vi "VISA GPIB Write-Read.vi"(5 "Max Bytes":u32=8000, 6 "Wait For SRQ":bool, 7 "Wait (ms)":u32, 8 "error in (no error)":errorcluster {"code" format="%.0x"}, 9 "Command":string, 10 "Action":enum16{"Write", "Read", "Write & Read"}(ring), 11 "VISA resource name":refnum<visa-resource-name>) -> (0 "error out":errorcluster {"code" format="%.0x"}, 1 "Read ∆ Time":dbl format="%.4f", 2 "String Returned":string, 3 "dup VISA Session":refnum<visa-resource-name>)   [LabVIEW 2024]
doc: "Does a write, read or an uninterrupted write/read since not reentrant. Locks the VISA resource to keep from being interfered with.\nAction: 0=Write, 1=Read, 2=Write followed by Read\nThe read portion is modifed to deal with Oxford's use of carriage returns rather than EOI\nScott Hannahs, <sth@magnet.fsu.edu> NHMFL-FSU, May 2003"
uses:
  <vilib>/Instr/_visa.llb/Select Event Type.ctl
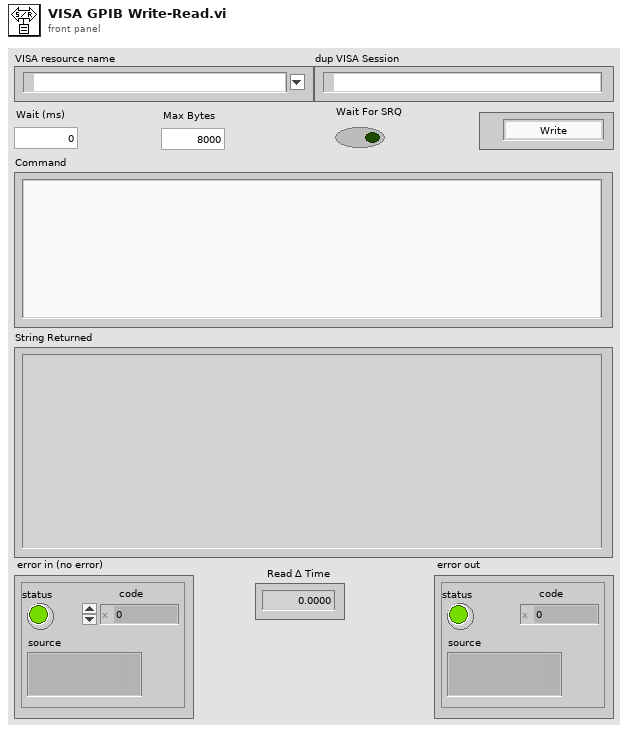
[diagram p1: front panel]
types:
  T1 = typedef "Select Event Type.ctl" = u32
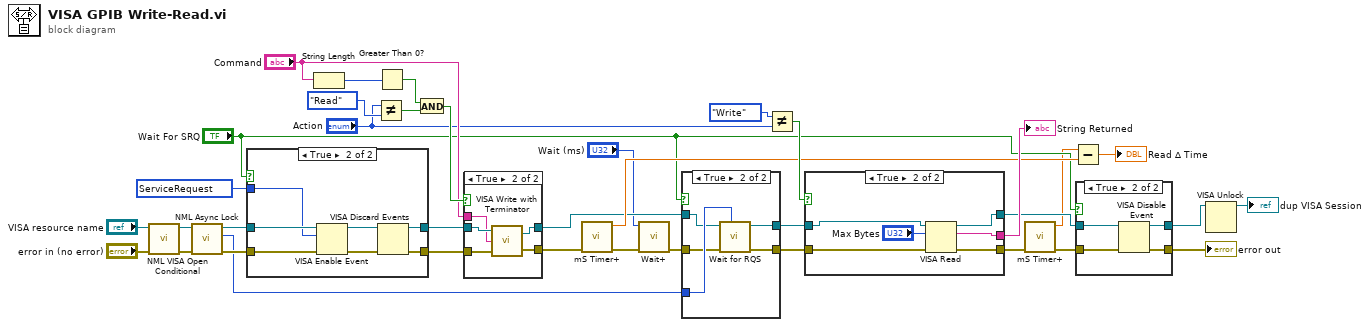
[diagram p0: block diagram]
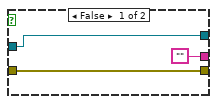
[diagram p5: hidden frame]
diagram:
  w16 = T1 1073684491 items=["ServiceRequest"=1073684491, "Trigger"=3221168138, "Clear"=1073684493, "VXI-Signal"=1073684512, "VXI/VME-Interrupt"=3221168161, "VXI/VME-Sysfail"=1073684509, "VXI/VME-Sysreset"=1073684510, "GPIB-CIC"=1073684498, "GPIB-Talk"=1073684499, "GPIB-Listen"=1073684500, "PXI-Interrupt"=1073684514, "Serial-Break"=1073684515, "Serial-TermChar"=1073684516, "Serial-CTS"=1073684521, "Serial-DSR"=1073684522, "Serial-DCD"=1073684524, "Serial-RI"=1073684526, "Serial-Character"=1073684533, "USB-Interrupt"=1073684535, "AllEnabled"=1073709055] ("Event Type")
  n1 = call "NML VISA Open Conditional.vi"("error in (no error)"="error in (no error)", "VISA resource name"="VISA resource name") -> ("error out"=w9:errorcluster, "dup VISA Session"=w10:refnum<visa-resource-name>)  [unwired: 7 in, 1 out]
  n2 = call "NML Async Lock.vi"("error in (no error)"=w9, "VISA Refnum in"=w10) -> ("error out"=w19:errorcluster, "Timeout"=w11:u32, "VISA Refnum out"=w20:refnum<visa-resource-name>)  [unwired: 7 in]
  n3 = case shown="True" "Wait For SRQ" {
    tunnel: w20 -> [w39 w44]
    tunnel: w19 -> [w38 w43]
    tunnel: [w39 w42] -> w18
    tunnel: [w38 w41] -> w17
    tunnel: w16 -> [_ w40]
    frame False {
    }
    frame True {
      n4 = VISA Enable Event(8:w43, 10:w40, 11:w44) -> (0:w46:errorcluster, 3:w45:refnum<visa-resource-name>)  [unwired: 1 in]
      n5 = VISA Discard Events(8:w46, 11:w45) -> (0:w41:errorcluster, 3:w42:refnum<visa-resource-name>)  [unwired: 2 in]
    }
  }
  n6 = String Length(string="Command") -> (length=w33:i32)
  n7 = Not Equal?(x="Action", y=enum16{"Write", "Read", "Write & Read"}."Read") -> (x != y?=w36:bool)
  n8 = Greater Than 0?(x=w33) -> (x > 0?=w32:bool)
  n9 = And(x=w32, y=w36) -> (x .and. y?=w34:bool)
  n10 = case shown="True" w34 {
    tunnel: [w48 w53] -> w26
    tunnel: w17 -> [w48 w50]
    tunnel: "Command" -> [_ w49]
    tunnel: [w47 w52] -> w6
    tunnel: w18 -> [w47 w51]
    frame False {
    }
    frame True {
      n11 = call "VISA Write with Terminator.vi"("error in (no error)"=w50, "String to Write"=w49, "VISA session"=w51) -> ("error out"=w53:errorcluster, "dup VISA session"=w52:refnum<visa-resource-name>)
    }
  }
  n12 = call "mS Timer+.vi"("Error In"=w26) -> ("Error Out"=w4:errorcluster, "MilliSecond Timer Value"=w25:dbl)  [unwired: 9 in]
  n13 = call "Wait+.vi"("Error In"=w4, "milliseconds to wait"="Wait (ms)") -> ("Error Out"=w5:errorcluster)  [unwired: 4 in, 1 out]
  n14 = case shown="True" "Wait For SRQ" {
    tunnel: w6 -> [w55 w56]
    tunnel: [w55 w60] -> w22
    tunnel: [w54 w59] -> w21
    tunnel: w5 -> [w54 w57]
    tunnel: w11 -> [_ w58]
    frame False {
    }
    frame True {
      n15 = call <vilib>:"Wait for RQS.VI"("timeout (25000 ms)"=w58, "error in (no error)"=w57, "VISA resource name"=w56) -> ("error out"=w59:errorcluster, "VISA resource name out"=w60:refnum<visa-resource-name>)  [unwired: 6 in, 1 out]
    }
  }
  n16 = Not Equal?(x=enum16{"Write", "Read", "Write & Read"}."Write" ("y"), y="Action") -> (x != y?=w35:bool)
  n17 = case shown="True" w35 {
    tunnel: [w63 w66] -> w27
    tunnel: w21 -> [w63 w69]
    tunnel: w22 -> [w61 w68]
    tunnel: ["" w67] -> w28
    tunnel: [w61 w65] -> w24
    frame False {
    }
    frame True {
      n18 = VISA Read(VISA resource name=w68, byte count="Max Bytes", error in (no error)=w69) -> (VISA resource name out=w65:refnum<visa-resource-name>, read buffer=w67:string, error out=w66:errorcluster)  [unwired: 1 out]
    }
  }
  "String Returned" <- w28
  n19 = call "mS Timer+.vi"("Error In"=w27) -> ("Error Out"=w13:errorcluster, "MilliSecond Timer Value"=w1:dbl)  [unwired: 9 in]
  n20 = Subtract(x=w1, y=w25) -> (x-y=→"Read ∆ Time":dbl)
  n21 = case shown="True" "Wait For SRQ" {
    tunnel: [w71 w75] -> w15
    tunnel: [w70 w74] -> w14
    tunnel: w13 -> [w70 w73]
    tunnel: w24 -> [w71 w72]
    frame False {
    }
    frame True {
      n22 = VISA Disable Event(8:w73, 11:w72) -> (0:w74:errorcluster, 3:w75:refnum<visa-resource-name>)  [unwired: 2 in]
    }
  }
  "error out" <- w14
  n23 = VISA Unlock(11:w15) -> (3:→"dup VISA Session":refnum<visa-resource-name>)  [unwired: 1 in, 1 out]
